vi "IsLeftTunnel__slk_mt.vi"(8 "error in (no error)":errorcluster, 11 "tunnel refnum in":refnum<vi>) -> (0 "error out":errorcluster, 2 "left tunnel?":bool, 3 "duplicated tunnel refnum out":refnum<vi>)   [LabVIEW 2013, in "Lazyboots Menu Tool.lvlib"]
doc: "Checks if the tunnel is at left."
uses:
  Library/Lazyboots Menu Tool.lvlib
panel:
  # "IsLeftTunnel__slk_mt.vi\nChecks if the tunnel is at left.\n\nNOTICE -- YOU MUST LEAVE THIS NOTICE IN PLACE.\n\nCopyright (c) 2011, LIANG LIU Shawn.Liu.cn@gmail.com\nAll rights reserved.\n\nRedistribution and use in source and binary forms, with or without modification, are permitted provided that the following conditions are met:\n-Redistributions of source code must retain the above copyright notice, this list of conditions and the following disclaimer.\n-Redistributions in binary form must reproduce the above copyright notice, this list of conditions and the following disclaimer in the documentation and/or other materials provided with the distribution.\n-Neither the name of the eLp nor the names of its contributors may be used to endorse or promote products derived from this software without specific prior written permission.\n\nTHIS SOFTWARE IS PROVIDED BY THE COPYRIGHT HOLDERS AND CONTRIBUTORS \"AS IS\" AND ANY EXPRESS OR IMPLIED WARRANTIES, INCLUDING, BUT NOT LIMITED TO, THE IMPLIED WARRANTIES OF MERCHANTABILITY AND FITNESS FOR A PARTICULAR PURPOSE ARE DISCLAIMED. IN NO EVENT SHALL THE COPYRIGHT HOLDER OR CONTRIBUTORS BE LIABLE FOR ANY DIRECT, INDIRECT, INCIDENTAL, SPECIAL, EXEMPLARY, OR CONSEQUENTIAL DAMAGES (INCLUDING, BUT NOT LIMITED TO, PROCUREMENT OF SUBSTITUTE GOODS OR SERVICES; LOSS OF USE, DATA, OR PROFITS; OR BUSINESS INTERRUPTION) HOWEVER CAUSED AND ON ANY THEORY OF LIABILITY, WHETHER IN CONTRACT, STRICT LIABILITY, OR TORT (INCLUDING NEGLIGENCE OR OTHERWISE) ARISING IN ANY WAY OUT OF THE USE OF THIS SOFTWARE, EVEN IF ADVISED OF THE POSSIBILITY OF SUCH DAMAGE."
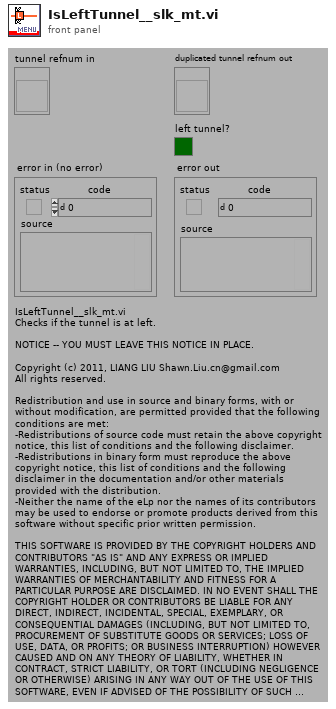
[diagram p1: front panel]
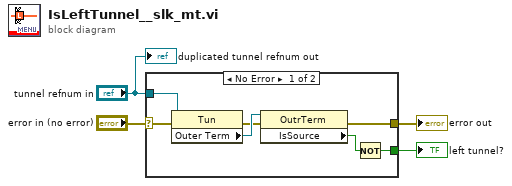
[diagram p0: block diagram]
diagram:
  n1 = case shown="No Error" "error in (no error)" {
    selector: "error in (no error)" -> [w9 w13]
    tunnel: [w5 FALSE] -> w4
    tunnel: [w7 w13] -> w3
    tunnel: "tunnel refnum in" -> [w8 _]
    frame No Error {
      n2 = property class="Tun"(reference=w8, error in=w9) -> (error out=w10:errorcluster, "Outer Term"=w11:refnum<vi>)  [unwired: 1 out]
      n3 = property class="OutrTerm"(reference=w11, error in=w10) -> (error out=w7:errorcluster, "IsSource"=w6:bool)  [unwired: 1 out]
      n4 = Not(x=w6) -> (.not. x?=w5:bool)
    }
    frame Error {
    }
  }
  "left tunnel?" <- w4
  "error out" <- w3
  "duplicated tunnel refnum out" <- "tunnel refnum in"
